vi "Index Array - Checked.vi"   [LabVIEW 2018, in "Utilities.lvlib"]
uses:
  Utilities.lvlib
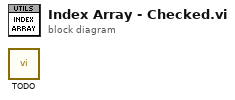
[diagram p0: block diagram]
diagram:
  n1 = call "TODO.vi"() -> ()  [unwired: 12 in]
